vi "PSRR Test.vi"(0 "TSM context":T1, 1 "Capture Time (s)":dbl=1.0 format="%#_13g", 5 "Vdd Voltage":dbl=2.8 format="%#_13g", 7 "Sine Ripple Vpp (V)":dbl=0.1 format="%#_13g", 9 "Sine Ripple Frequency (Hz)":dbl=1000.0 format="%#_13g") -> (15 "error out":errorcluster)   [LabVIEW 2020]
doc: "VI calculates PSRR(In dB) by powering the DUT with input DC signal with AC ripples (Vpp) at a specific frequency and measures the equivalent microphone output Vpp at the same frequency under no stimilus and obtains the ratio in dB range."
uses:
  <vilib>/NI_TestStand_SemiconductorModule/NI_TestStand_Semiconductor_Module.lvlibp/PinMap/General/SemiconductorModuleContext.ctl
  <vilib>/NI_TestStand_SemiconductorModule/NI_TestStand_Semiconductor_Module.lvlibp/PinMap/TagProvider/TSM_Pin.ctl
  46e31d67-da63-4e09-af4c-2002d0e6ed37.vi
  e83f53a7-dc9a-466a-a226-fadaa6e6d0a3.vi
  <vilib>/measure/matone.llb/Extract Single Tone Information N Chan.vi
  <vilib>/NI_TestStand_SemiconductorModule/NI_TestStand_Semiconductor_Module.lvlibp/PinMap/General/Publish/PublishDataDoubleFunctionalTest.vi
  <vilib>/NI_TestStand_SemiconductorModule/NI_TestStand_Semiconductor_Module.lvlibp
  <vilib>/measure/NI_MABase.lvlib
  <vilib>/measure/NI_MAPro.lvlib
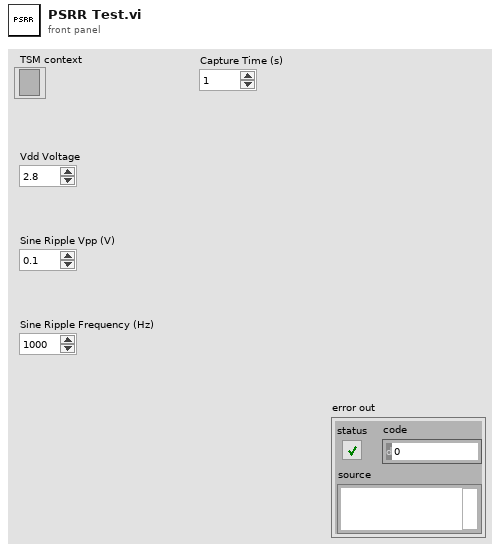
[diagram p1: front panel]
types:
  T1 = typedef "NI_TestStand_Semiconductor_Module.lvlibp/SemiconductorModuleContext.ctl" = refnum<k7>
  T2 = typedef "NI_TestStand_Semiconductor_Module.lvlibp/TSM_Pin.ctl" = tag
  T3 = cluster{"approx freq. (optional)":dbl, "search (+/- % of Fsampl.)":dbl}
  T4 = typedef "TSM DAQmx Multi-Task.ctl" = cluster{"Pin Query Context":refnum<class "MultiplePinMultipleSessionQueryContext.lvclass">, "SSC":T5[], "Site Numbers":i32[], "Pins":tag[]}
  T5 = typedef "SSC DAQmx.ctl" = cluster{"DAQmx Task ":refnum<k21>, "Channels":string, "Channel Lists":string}
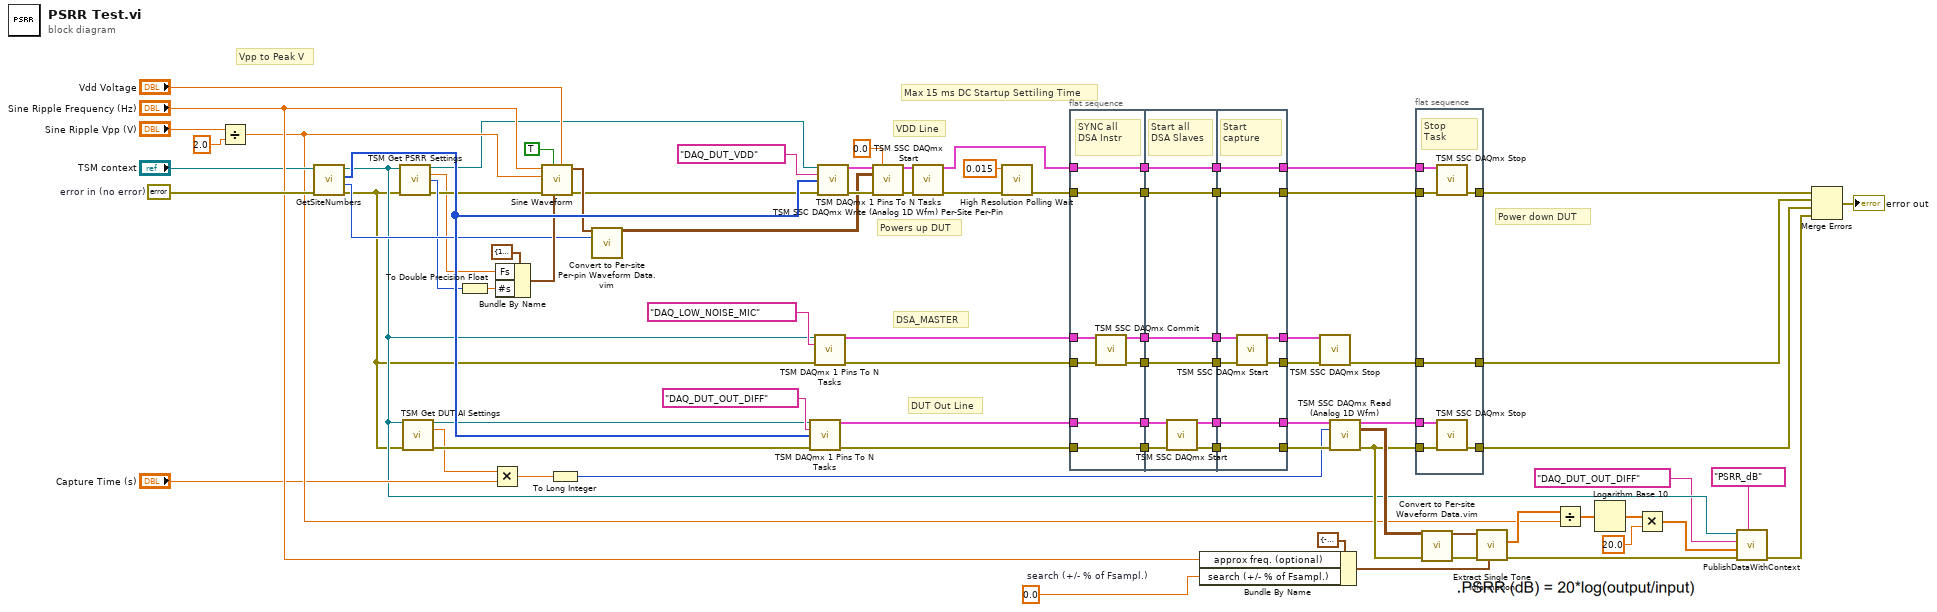
[diagram p0: block diagram]
diagram:
  w46 = 0.0  # search (+/- % of Fsampl.)
  w83 = errorcluster {"status"=FALSE, "code"=0, "source"=""}  # error in (no error)
  # "DSA_MASTER"
  # "Max 15 ms DC Startup Settiling Time"
  # "Vpp to Peak V"
  # "DUT Out Line"
  # "VDD Line"
  # "Power down DUT"
  # "Powers up DUT"
  n1 = Divide(x="Sine Ripple Vpp (V)", y=2.0 ("x")) -> (x/y=w38:dbl)
  n2 = call <vilib>:"GetSiteNumbers.vi"("error in (no error)"=w83, "Semiconductor Module Context"="TSM context") -> ("error out"=w5:errorcluster, "Number Of Sites"=w63:i32, "Site Numbers"=w80:i32[], "Semiconductor Module Context Out"=w6:T1)  [unwired: 6 in]
  n3 = call "TSM Get PSRR Settings.vi"("TSM context"=w6, "error in (no error)"=w5) -> ("TSM context Out"=w28:T1, "Sampling Rate (Hz)"=w32:dbl, "Samples per channel"=w56:i32, "error out"=w39:errorcluster)  [unwired: 8 in, 2 out]
  n4 = call "TSM Get DUT AI Settings.vi"("TSM context"=w6, "error in (no error)"=w5) -> ("TSM context Out"=w4:T1, "Sampling Rate (Hz)"=w2:dbl, "error out"=w3:errorcluster)  [unwired: 9 in, 2 out]
  n5 = To Double Precision Float(number=w56) -> (double precision float=w76:dbl)
  n6 = Multiply(x=w2, y="Capture Time (s)") -> (x*y=w30:dbl)
  n7 = Bundle By Name(cluster=cluster{"Fs":dbl, "#s":dbl} {"Fs"=1000.0, "#s"=1000.0} ("sampling info"), "Fs"=w32, "#s"=w76) -> (w75:cluster{"Fs":dbl, "#s":dbl})
  n8 = call <vilib>:"Sine Waveform.vi"("offset"="Vdd Voltage", "sampling info"=w75, "reset signal"=TRUE, "error in (no error)"=w39, "amplitude"=w38, "frequency"="Sine Ripple Frequency (Hz)") -> ("error out"=w27:errorcluster, "signal out"=w62:waveform(dbl))  [unwired: 4 in]
  n9 = To Long Integer(number=w30) -> (32bit integer=w33:i32)
  n10 = call "Convert to Per-site Per-pin Waveform Data.vim"("Waveform In"=w62, "No. of Site"=w63) -> ("Per Site Per Pin Waveform Out"=w61:waveform(dbl)[][])  [unwired: 13 in]
  n11 = call "TSM DAQmx 1 Pins To N Tasks.vi"("TSM context"=w4, "Pins"=tag "DAQ_DUT_OUT_DIFF", "Site Numbers"=w80, "error in"=w3) -> ("DAQ TSM Out"=w71:T4, "error out"=w72:errorcluster)  [unwired: 10 in]
  n12 = call "TSM DAQmx 1 Pins To N Tasks.vi"("TSM context"=w6, "Pins"=tag "DAQ_LOW_NOISE_MIC", "error in"=w5) -> ("DAQ TSM Out"=w21:T4, "error out"=w22:errorcluster)  [unwired: 11 in]
  n13 = call "TSM DAQmx 1 Pins To N Tasks.vi"("TSM context"=w28, "Pins"=tag "DAQ_DUT_VDD", "Site Numbers"=w80, "error in"=w27) -> ("DAQ TSM Out"=w73:T4, "error out"=w79:errorcluster)  [unwired: 10 in]
  n14 = call "TSM SSC DAQmx Write (Analog 1D Wfm) Per-Site Per-Pin.vi"("DAQ TSM in"=w73, "Idle Channel Value (0)"=0.0, "Per-Site Per-Pin Waveforms in"=w61, "error in"=w79) -> ("DAQ TSM Out"=w60:T4, "error out"=w64:errorcluster)  [unwired: 10 in]
  n15 = call "TSM SSC DAQmx Start.vi"("TSM DAQmx In"=w60, "error in (no error)"=w64) -> ("TSM DAQmx Out"=w67:T4, "error out"=w70:errorcluster)  [unwired: 12 in]
  n16 = call <vilib>:"High Resolution Polling Wait.vi"("error in (no error)"=w70, "seconds to wait"=0.015) -> ("error out"=w68:errorcluster)  [unwired: 9 in]
  n17 = flat-sequence {
    tunnel: w67 -> [w88]
    tunnel: w68 -> [w89]
    tunnel: w71 -> [w90]
    tunnel: w72 -> [w91]
    tunnel: [w91] -> w26
    tunnel: [w90] -> w25
    tunnel: [w89] -> w24
    tunnel: [w88] -> w23
    tunnel: w22 -> [w87]
    tunnel: w21 -> [w86]
    tunnel: [w85] -> w20
    tunnel: [w84] -> w19
    tunnel: w26 -> [w99]
    tunnel: w25 -> [w98]
    tunnel: w24 -> [w97]
    tunnel: w23 -> [w96]
    tunnel: w20 -> [w93]
    tunnel: w19 -> [w92]
    tunnel: [w97] -> w18
    tunnel: [w96] -> w17
    tunnel: [w95] -> w16
    tunnel: [w94] -> w15
    tunnel: [w93] -> w14
    tunnel: [w92] -> w13
    tunnel: [w104] -> w59
    tunnel: [w105] -> w58
    tunnel: [w106] -> w66
    tunnel: [w107] -> w65
    tunnel: w18 -> [w107]
    tunnel: w17 -> [w106]
    tunnel: w16 -> [w105]
    tunnel: w15 -> [w104]
    tunnel: w14 -> [w102]
    tunnel: w13 -> [w103]
    tunnel: [w101] -> w11
    tunnel: [w100] -> w12
    frame #0 {
      # "SYNC all DSA Instr"
      n18 = call "TSM SSC DAQmx Commit.vi"("TSM DAQmx In"=w86, "error in (no error)"=w87) -> ("TSM DAQmx Out"=w85:T4, "error out"=w84:errorcluster)  [unwired: 12 in]
    }
    frame #1 {
      # "Start all DSA Slaves"
      n19 = call "TSM SSC DAQmx Start.vi"("TSM DAQmx In"=w98, "error in (no error)"=w99) -> ("TSM DAQmx Out"=w94:T4, "error out"=w95:errorcluster)  [unwired: 12 in]
    }
    frame #2 {
      # "Start capture"
      n20 = call "TSM SSC DAQmx Start.vi"("TSM DAQmx In"=w102, "error in (no error)"=w103) -> ("TSM DAQmx Out"=w101:T4, "error out"=w100:errorcluster)  [unwired: 12 in]
    }
  }
  n21 = Bundle By Name(cluster=T3 {"approx freq. (optional)"=-1.0, "search (+/- % of Fsampl.)"=5.0} ("advanced search"), "approx freq. (optional)"="Sine Ripple Frequency (Hz)", "search (+/- % of Fsampl.)"=w46) -> (w45:T3)
  n22 = call "TSM SSC DAQmx Stop.vi"("TSM DAQmx In"=w11, "error in (no error)"=w12) -> ("error out"=w10:errorcluster)  [unwired: 12 in, 1 out]
  n23 = call "TSM SSC DAQmx Read (Analog 1D Wfm).vi"("DAQ TSM in"=w59, "Samples to read"=w33, "error in"=w58) -> ("DAQ TSM Out"=w57:T4, "Per-Site Per-Pin Waveforms Out"=w55:waveform(dbl)[][], "error out"=w51:errorcluster)  [unwired: 10 in]
  n24 = flat-sequence {
    tunnel: w66 -> [w114]
    tunnel: w65 -> [w113]
    tunnel: w57 -> [w112]
    tunnel: w51 -> [w111]
    tunnel: [w110] -> w9
    tunnel: [w109] -> w54
    tunnel: [w108] -> w8
    tunnel: w10 -> [w108]
    frame #0 {
      # "Stop \nTask"
      n25 = call "TSM SSC DAQmx Stop.vi"("TSM DAQmx In"=w114, "error in (no error)"=w113) -> ("error out"=w109:errorcluster)  [unwired: 12 in, 1 out]
      n26 = call "TSM SSC DAQmx Stop.vi"("TSM DAQmx In"=w112, "error in (no error)"=w111) -> ("error out"=w110:errorcluster)  [unwired: 12 in, 1 out]
    }
  }
  n27 = call "Convert to Per-site Waveform Data.vim"("Per-Site Per-Pin Waveform In"=w55) -> ("Per-Site Waveform Out"=w52:waveform(dbl)[])  [unwired: 14 in]
  n28 = call-poly <vilib>:"Extract Single Tone Information.vi"("advanced search"=w45, "error in (no error)"=w51, "time signals in"=w52) -> ("error out"=w44:errorcluster, "detected amplitudes"=w50:dbl[])  [unwired: 3 in, 4 out]
  n29 = Divide(x=w50, y=w38) -> (x/y=w36:dbl[])
  n30 = Logarithm Base 10(1:w36) -> (0:w35:dbl[])
  n31 = Multiply(x=w35, y=20.0) -> (x*y=w42:dbl[])
  n32 = call-poly <vilib>:"PublishDataWithContext.vi"("Published Data Id"=tag "PSRR_dB", "error in (no error)"=w44, "Data In"=w42, "Pin"=T2 "DAQ_DUT_OUT_DIFF", "Semiconductor Module Context"=w6) -> ("error out"=w41:errorcluster)  [unwired: 5 in, 1 out]
  n33 = Merge Errors(w54, w8, w9, w41) -> (→"error out":errorcluster)
